vi "fault and error bookkeeping.vi"(0 "data table in":T10, 1 "fault fifo":refnum<k33>, 2 "worker pool reference":T2, 5 "module data":T5={"run state"=enum."sync", "module"=refnum, "module ref"=refnum, "async exec ref"={"command fifo"=refnum, "error fifo"=refnum, "VI Refnum"=refnum, "input buffer"=refnum, "output buffer"=refnum, "process buffer"=refnum, "original dvrs"=[]}, "configuration ref"=refnum, "GUID"={"Hi"=0, "Lo"=0}, "error"={"status"=FALSE, "code"=0, "source"=""}, "previous error code"=0, "input method"={"data table"={"Double"=[], "Single"=[], "I64"=[], "I32"=[], "I16"=[], "I8"=[], "U64"=[], "U32"=[], "U16"=[], "U8"=[], "Boolean"=[], "String"=[], "Array of Double"=[], "Array of Single"=[], "Array of I64"=[], "Array of I32"=[], "Array of I16"=[], "Array of I8"=[], "Array of U64"=[], "Array of U32"=[], "Array of U16"=[], "Array of U8"=[], "Array of Boolean"=[], "Array of String"=[]}, "transfer spec"=[]}, "output method"={"data table"={"Double"=[], "Single"=[], "I64"=[], "I32"=[], "I16"=[], "I8"=[], "U64"=[], "U32"=[], "U16"=[], "U8"=[], "Boolean"=[], "String"=[], "Array of Double"=[], "Array of Single"=[], "Array of I64"=[], "Array of I32"=[], "Array of I16"=[], "Array of I8"=[], "Array of U64"=[], "Array of U32"=[], "Array of U16"=[], "Array of U8"=[], "Array of Boolean"=[], "Array of String"=[]}, "transfer spec"=[]}, "process method parameters"={"data table"={"Double"=[], "Single"=[], "I64"=[], "I32"=[], "I16"=[], "I8"=[], "U64"=[], "U32"=[], "U16"=[], "U8"=[], "Boolean"=[], "String"=[], "Array of Double"=[], "Array of Single"=[], "Array of I64"=[], "Array of I32"=[], "Array of I16"=[], "Array of I8"=[], "Array of U64"=[], "Array of U32"=[], "Array of U16"=[], "Array of U8"=[], "Array of Boolean"=[], "Array of String"=[]}, "transfer spec"=[]}, "process method results"={"data table"={"Double"=[], "Single"=[], "I64"=[], "I32"=[], "I16"=[], "I8"=[], "U64"=[], "U32"=[], "U16"=[], "U8"=[], "Boolean"=[], "String"=[], "Array of Double"=[], "Array of Single"=[], "Array of I64"=[], "Array of I32"=[], "Array of I16"=[], "Array of I8"=[], "Array of U64"=[], "Array of U32"=[], "Array of U16"=[], "Array of U8"=[], "Array of Boolean"=[], "Array of String"=[]}, "transfer spec"=[]}, "fault handling"={"unknown"=[], "trivial"=[], "critical"=[], "recoverable"=[]}, "error report index "=-1} {"GUID"."Lo" format="%.0x"; "GUID"."Hi" format="%.0x"}, 7 "time data in":T1, 9 "run flags in":u8, 11 "engine error in":errorcluster, 12 "module index":i32) -> (4 "data table out":T10, 6 "module data out":T5={"run state"=enum."sync", "module"=refnum, "module ref"=refnum, "async exec ref"={"command fifo"=refnum, "error fifo"=refnum, "VI Refnum"=refnum, "input buffer"=refnum, "output buffer"=refnum, "process buffer"=refnum, "original dvrs"=[]}, "configuration ref"=refnum, "GUID"={"Hi"=0, "Lo"=0}, "error"={"status"=FALSE, "code"=0, "source"=""}, "previous error code"=0, "input method"={"data table"={"Double"=[], "Single"=[], "I64"=[], "I32"=[], "I16"=[], "I8"=[], "U64"=[], "U32"=[], "U16"=[], "U8"=[], "Boolean"=[], "String"=[], "Array of Double"=[], "Array of Single"=[], "Array of I64"=[], "Array of I32"=[], "Array of I16"=[], "Array of I8"=[], "Array of U64"=[], "Array of U32"=[], "Array of U16"=[], "Array of U8"=[], "Array of Boolean"=[], "Array of String"=[]}, "transfer spec"=[]}, "output method"={"data table"={"Double"=[], "Single"=[], "I64"=[], "I32"=[], "I16"=[], "I8"=[], "U64"=[], "U32"=[], "U16"=[], "U8"=[], "Boolean"=[], "String"=[], "Array of Double"=[], "Array of Single"=[], "Array of I64"=[], "Array of I32"=[], "Array of I16"=[], "Array of I8"=[], "Array of U64"=[], "Array of U32"=[], "Array of U16"=[], "Array of U8"=[], "Array of Boolean"=[], "Array of String"=[]}, "transfer spec"=[]}, "process method parameters"={"data table"={"Double"=[], "Single"=[], "I64"=[], "I32"=[], "I16"=[], "I8"=[], "U64"=[], "U32"=[], "U16"=[], "U8"=[], "Boolean"=[], "String"=[], "Array of Double"=[], "Array of Single"=[], "Array of I64"=[], "Array of I32"=[], "Array of I16"=[], "Array of I8"=[], "Array of U64"=[], "Array of U32"=[], "Array of U16"=[], "Array of U8"=[], "Array of Boolean"=[], "Array of String"=[]}, "transfer spec"=[]}, "process method results"={"data table"={"Double"=[], "Single"=[], "I64"=[], "I32"=[], "I16"=[], "I8"=[], "U64"=[], "U32"=[], "U16"=[], "U8"=[], "Boolean"=[], "String"=[], "Array of Double"=[], "Array of Single"=[], "Array of I64"=[], "Array of I32"=[], "Array of I16"=[], "Array of I8"=[], "Array of U64"=[], "Array of U32"=[], "Array of U16"=[], "Array of U8"=[], "Array of Boolean"=[], "Array of String"=[]}, "transfer spec"=[]}, "fault handling"={"unknown"=[], "trivial"=[], "critical"=[], "recoverable"=[]}, "error report index "=-1} {"GUID"."Lo" format="%.0x"; "GUID"."Hi" format="%.0x"}, 8 "safe state?":bool, 10 "run flags out":u8, 15 "engine error out":errorcluster)   [LabVIEW 2013, in "main engine.lvlib"]
uses:
  main engine/main engine.lvlib
  rt fault.ctl
  <vilib>/NI/Tag Bus Module Framework/runtime/error classification.ctl
  <vilib>/NI/Tag Bus Module Framework/module configuration/TBM module configuration.lvclass
  <vilib>/NI/Tag Bus/table/data table.ctl
  full module data.ctl
  <vilib>/NI/Tag Bus Module Framework/runtime/TBM module execution interface.lvclass
  module run state.ctl
  async executor/asynchronous executor reference.ctl
  async executor/message to executor.ctl
  async command notification.ctl
  async error info.ctl
  <vilib>/NI/Configuration Framework/serializable configuration/Numeric GUID.ctl
  module method data.ctl
  <vilib>/NI/Tag Bus/table/transfer specification.ctl
  <vilib>/NI/Tag Bus/tag/Data Type.ctl
  fault handling spec.ctl
  Configuration/Error Actions.ctl
  worker library/worker comms.ctl
  worker library/worker commands.ctl
  worker library/request fifos.ctl
  worker library/recovery request.ctl
  worker library/response fifos.ctl
  worker library/recovery response.ctl
  time information.ctl
  <vilib>/NI/Tag Bus/table/data polymorphs/write one/write I32.vi
  worker library/request recovery.vi
  rt swap object in dvr.vi
  <vilib>/NI/Tag Bus/table/data table.lvlib
  async executor/async executor.lvlib
  <vilib>/NI/Configuration Framework/serializable configuration/NISE_CEF_serializable configuration.lvclass
  Configuration/Standard Engine Configuration.lvclass
  <vilib>/NI/Tag Bus/tag/tag descriptor.lvclass
  worker library/worker pool.lvlib
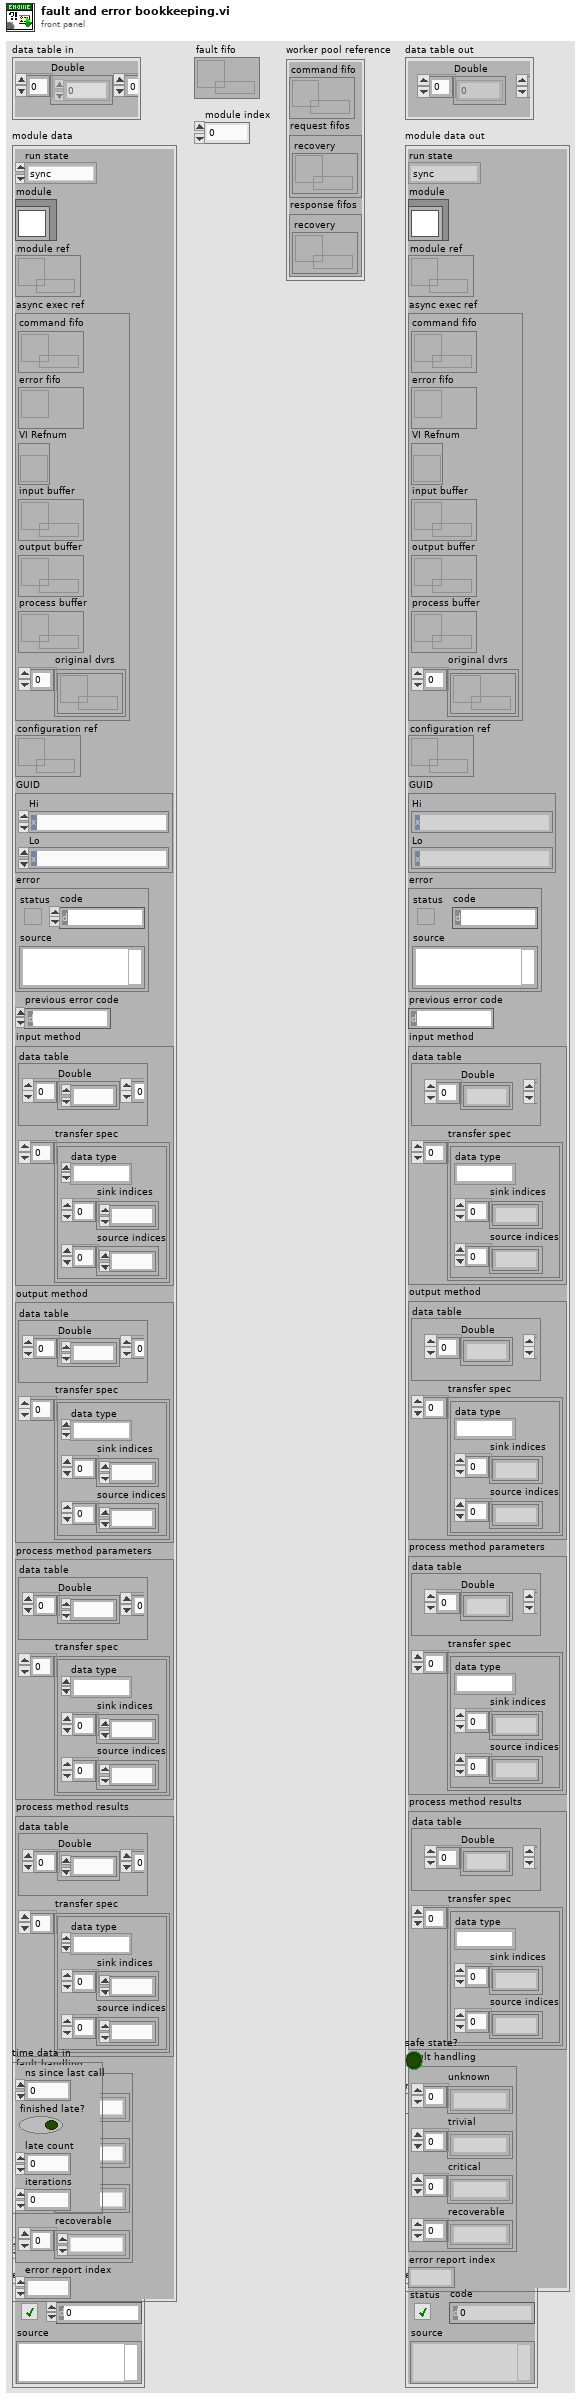
[diagram p1: front panel]
types:
  T1 = typedef "main engine.lvlib/time information.ctl" = cluster{"ns since last call":u64, "finished late?":bool, "late count":u32, "iterations":u64}
  T2 = typedef "worker pool.lvlib/worker comms.ctl" = cluster{"command fifo":refnum<k33>, "request fifos":T3, "response fifos":T4}
  T3 = typedef "worker pool.lvlib/request fifos.ctl" = cluster{"recovery":refnum<k33>}
  T4 = typedef "worker pool.lvlib/response fifos.ctl" = cluster{"recovery":refnum<k33>}
  T5 = typedef "main engine.lvlib/full module data.ctl" = cluster{"run state":T6, "module":refnum<class "TBM module execution interface.lvclass">, "module ref":refnum<data-value>, "async exec ref":T7, "configuration ref":refnum<data-value>, "GUID":T8, "error":errorcluster, "previous error code":i32, "input method":T9, "output method":T9, "process method parameters":T9, "process method results":T9, "fault handling":T13, "error report index ":i32}
  T6 = typedef "main engine.lvlib/module run state.ctl" = enum16{"sync", "async"}
  T7 = typedef "async executor.lvlib/asynchronous executor reference.ctl" = cluster{"command fifo":refnum<k33>, "error fifo":refnum<k33>, "VI Refnum":refnum<vi>, "input buffer":refnum<k33>, "output buffer":refnum<k33>, "process buffer":refnum<k33>, "original dvrs":refnum<data-value>[]}
  T8 = typedef "NISE_CEF_serializable configuration.lvclass/Numeric GUID.ctl" = cluster{"Hi":u64, "Lo":u64}
  T9 = typedef "main engine.lvlib/module method data.ctl" = cluster{"data table":T10, "transfer spec":T11[]}
  T10 = typedef "tag bus.lvlib/data table.lvlib/data table.ctl" = cluster{"Double":dbl[], "Single":sgl[], "I64":i64[], "I32":i32[], "I16":i16[], "I8":i8[], "U64":u64[], "U32":u32[], "U16":u16[], "U8":u8[], "Boolean":bool[], "String":string[], "Array of Double":cluster{"DBL Array":dbl[]}[], "Array of Single":cluster{"SGL Array":sgl[]}[], "Array of I64":cluster{"I64 Array":i64[]}[], "Array of I32":cluster{"I32 Array":i32[]}[], "Array of I16":cluster{"I16 Array":i16[]}[], "Array of I8":cluster{"I8 Array":i8[]}[], "Array of U64":cluster{"U64 Array":u64[]}[], "Array of U32":cluster{"U32 Array":u32[]}[], "Array of U16":cluster{"U16 Array":u16[]}[], "Array of U8":cluster{"U8 Array":u8[]}[], "Array of Boolean":cluster{"Boolean Array":bool[]}[], "Array of String":cluster{"String Array":string[]}[]}
  T11 = typedef "tag bus.lvlib/data table.lvlib/transfer specification.ctl" = cluster{"data type":T12, "sink indices":i32[], "source indices":i32[]}
  T12 = typedef "tag bus.lvlib/tag descriptor.lvclass/Data Type.ctl" = enum16{"Double", "Single", "I64", "I32", "I16", "I8", "U64", "U32", "U16", "U8", "Boolean", "String", "Array of Double", "Array of Single", "Array of I64", "Array of I32", "Array of I16", "Array of I8", "Array of U64", "Array of U32", "Array of U16", "Array of U8", "Array of Boolean", "Array of String"}
  T13 = typedef "main engine.lvlib/fault handling spec.ctl" = cluster{"unknown":T14[], "trivial":T14[], "critical":T14[], "recoverable":T14[]}
  T14 = typedef "Standard Engine Configuration.lvclass/Error Actions.ctl" = enum16{"Clear", "Notify", "Stop Component", "Stop Engine", "Safe State", "Attempt Recovery"}
  T15 = typedef "TBM module execution interface.lvclass/error classification.ctl" = enum16{"unknown", "none", "trivial", "recoverable", "critical"}
  T16 = typedef "async executor.lvlib/async error info.ctl" = cluster{"error code":i32, "error classification":T15}
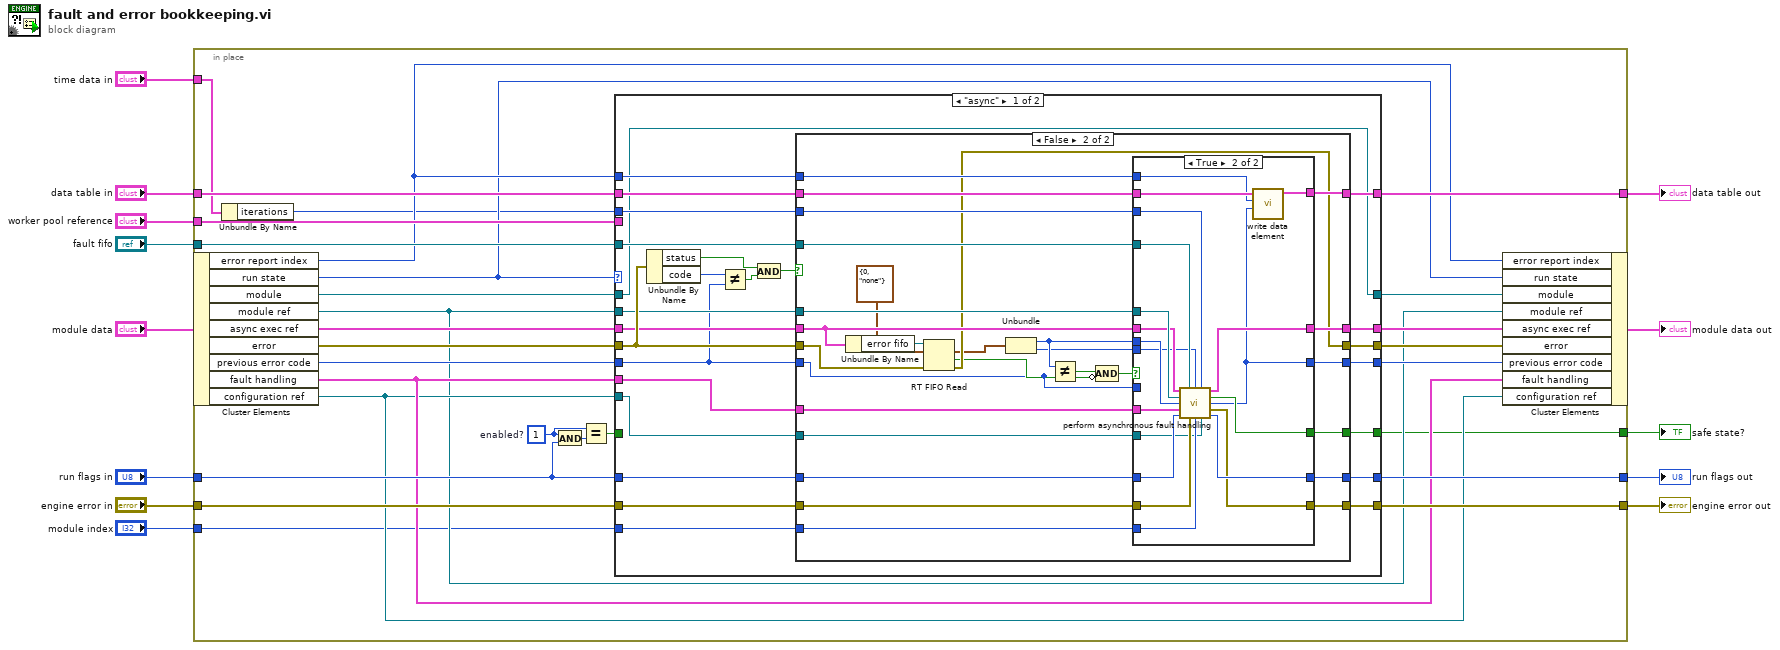
[diagram p0: block diagram]
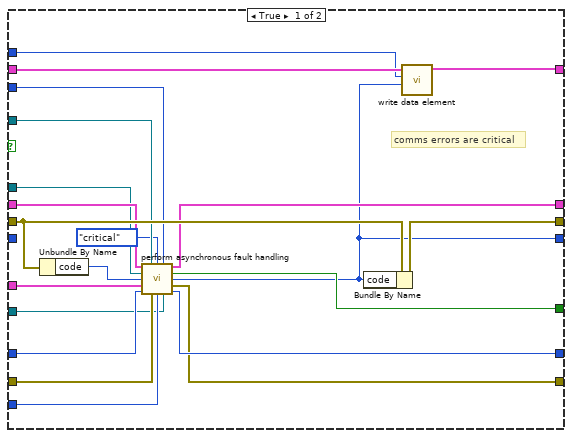
[diagram p2: hidden frame]
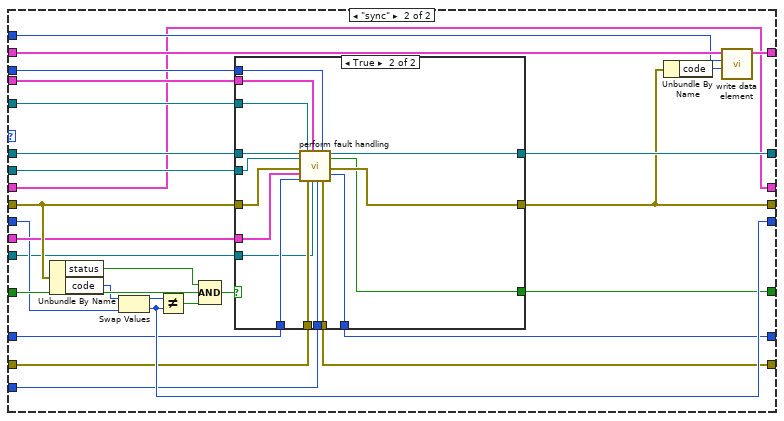
[diagram p4: hidden frame]
diagram:
  n1 = in-place {
    in-place-border: [w41] -> w13
    in-place-border: "run flags in" -> [w40]
    in-place-border: "fault fifo" -> [w39]
    in-place-border: [w35] -> w10
    in-place-border: "data table in" -> [w34]
    in-place-border: "engine error in" -> [w33]
    in-place-border: [w32] -> w7
    in-place-border: "worker pool reference" -> [w31]
    in-place-border: "time data in" -> [w17]
    in-place-border: "module index" -> [w16]
    in-place-border: [w14] -> w1
    w37 = u8 1  # enabled?
    n2 = in-place-cluster #1("module data") -> ("error report index"=w30:i32, "run state"=w29:T6, "module"=w28:refnum<class "TBM module execution interface.lvclass">, "module ref"=w18:refnum<data-value>, "async exec ref"=w27:T7, "error"=w26:errorcluster, "previous error code"=w25:i32, "fault handling"=w20:T13, "configuration ref"=w19:refnum<data-value>)
    n3 = Unbundle By Name(w17) -> ("iterations"=w15:u64)
    n4 = And(x=w37, y=w40) -> (x .and. y?=w36:u8)
    n5 = Equal?(x=w37, y=w36) -> (x = y?=w38:bool)
    n6 = case shown="\"async\"" w29 {
      tunnel: w34 -> [w65 w168]
      tunnel: [w64 w167] -> w35
      tunnel: w30 -> [w63 w166]
      tunnel: w38 -> [_ w165]
      tunnel: w28 -> [w42 w163]
      tunnel: [w42 w162] -> w21
      tunnel: [w59 w140] -> w22
      tunnel: w27 -> [w60 w140]
      tunnel: w26 -> [w61 w161]
      tunnel: w20 -> [w47 w160]
      tunnel: [w62 w150] -> w23
      tunnel: w18 -> [w50 w158]
      tunnel: w39 -> [w52 w157]
      tunnel: w25 -> [w43 w153]
      tunnel: [w58 w152] -> w24
      tunnel: [w57 w148] -> w41
      tunnel: w40 -> [w56 w149]
      tunnel: w33 -> [w55 w147]
      tunnel: [w49 w146] -> w32
      tunnel: w31 -> [_ w143]
      tunnel: w19 -> [w48 w145]
      tunnel: w16 -> [w54 w144]
      tunnel: w15 -> [w51 w142]
      tunnel: [w53 w141] -> w14
      frame "async" {
        n7 = Unbundle By Name(w61) -> ("status"=w66:bool, "code"=w44:i32)
        n8 = Not Equal?(x=w44, y=w43) -> (x != y?=w45:bool)
        n9 = And(x=w66, y=w45) -> (x .and. y?=w46:bool)
        n10 = case shown="False" w46 {
          tunnel: w65 -> [w86 w114]
          tunnel: [w87 w115] -> w64
          tunnel: w63 -> [w85 w113]
          tunnel: [w73 w97] -> w62
          tunnel: w61 -> [w84 w112]
          tunnel: w60 -> [w77 w98]
          tunnel: [w78 w106] -> w59
          tunnel: [w68 w99] -> w58
          tunnel: [w81 w109] -> w57
          tunnel: w56 -> [w80 w108]
          tunnel: w55 -> [w83 w111]
          tunnel: w54 -> [w82 w110]
          tunnel: [w79 w107] -> w53
          tunnel: w52 -> [w76 w105]
          tunnel: w51 -> [w75 w104]
          tunnel: w50 -> [w72 w103]
          tunnel: [w71 w102] -> w49
          tunnel: w48 -> [w70 w101]
          tunnel: w47 -> [w69 w100]
          tunnel: w43 -> [_ w92]
          frame True {
            # "comms errors are critical"
            n11 = Unbundle By Name(w84) -> ("code"=w74:i32)
            n12 = call "perform asynchronous fault handling.vi"("module in"=w77, "fault fifo"=w76, "error classification"=error_classification."critical", "iteration"=w75, "module ref in"=w72, "code"=w74, "fault handling in"=w69, "run flags in"=w80, "engine error in"=w83, "engine reference"=w82, "cfg ref"=w70) -> ("module out"=w78:T7, "go to safe state"=w79:bool, "code out"=w68:i32, "engine error out"=w71:errorcluster, "run flags out"=w81:u8)
            n13 = Bundle By Name(cluster=w84, "code"=w68) -> (w73:errorcluster)
            n14 = call-poly <vilib>:"write data element.vi"("value"=w68, "index"=w85, "data table in"=w86) -> ("data table out"=w87:T10)  [unwired: 8 in]
          }
          frame False {
            n15 = Unbundle By Name(w98) -> ("error fifo"=w96:refnum<k33>)
            n16 = RT FIFO Read(0:w96, 1:T16 {"error code"=0, "error classification"=enum."none"} ("element"), 3:w112) -> (9:w93:T16, 10:w95:bool, 11:w97:errorcluster)  [unwired: 1 in, 2 out]
            n17 = Unbundle(w93) -> ("error code"=w91:i32, "error classification"=w89:T15)
            n18 = Not Equal?(x=w91, y=w92) -> (x != y?=w90:bool)
            n19 = Compound Arithmetic op=AND(w90, invert w95) -> (w94:bool)
            n20 = case shown="True" w94 {
              tunnel: [w120 w139] -> w115
              tunnel: w114 -> [w120 w138]
              tunnel: w113 -> [_ w137]
              tunnel: w111 -> [w116 w136]
              tunnel: w110 -> [_ w135]
              tunnel: [w117 w134] -> w109
              tunnel: w108 -> [w117 w133]
              tunnel: [_ w132] -> w107
              tunnel: [w119 w131] -> w106
              tunnel: w105 -> [_ w130]
              tunnel: w104 -> [_ w129]
              tunnel: w103 -> [_ w128]
              tunnel: [w116 w127] -> w102
              tunnel: w101 -> [_ w126]
              tunnel: w100 -> [_ w125]
              tunnel: [w118 w124] -> w99
              tunnel: w98 -> [w119 w123]
              tunnel: w92 -> [w118 _]
              tunnel: w91 -> [_ w122]
              tunnel: w89 -> [_ w121]
              frame False {
              }
              frame True {
                n21 = call "perform asynchronous fault handling.vi"("module in"=w123, "fault fifo"=w130, "error classification"=w121, "iteration"=w129, "module ref in"=w128, "code"=w122, "fault handling in"=w125, "run flags in"=w133, "engine error in"=w136, "engine reference"=w135, "cfg ref"=w126) -> ("module out"=w131:T7, "go to safe state"=w132:bool, "code out"=w124:i32, "engine error out"=w127:errorcluster, "run flags out"=w134:u8)
                n22 = call-poly <vilib>:"write data element.vi"("value"=w124, "index"=w137, "data table in"=w138) -> ("data table out"=w139:T10)  [unwired: 8 in]
              }
            }
          }
        }
      }
      frame "sync" {
        n23 = Unbundle By Name(w161) -> ("status"=w159:bool, "code"=w154:i32)
        n24 = Swap Values(12:w154, 14:w153) -> (1:w155:i32, 3:w152:i32)  [unwired: 1 in]
        n25 = Not Equal?(x=w155, y=w152) -> (x != y?=w156:bool)
        n26 = Compound Arithmetic op=AND(w159, w165, w156) -> (w164:bool)
        n27 = case shown="True" w164 {
          tunnel: w163 -> [w172 w187]
          tunnel: [w172 w188] -> w162
          tunnel: w161 -> [w171 w183]
          tunnel: [w171 w185] -> w150
          tunnel: w160 -> [_ w184]
          tunnel: w158 -> [_ w186]
          tunnel: w157 -> [_ w180]
          tunnel: w149 -> [w170 w182]
          tunnel: [w170 w181] -> w148
          tunnel: w147 -> [w169 w179]
          tunnel: [w169 w178] -> w146
          tunnel: w145 -> [_ w177]
          tunnel: w144 -> [_ w176]
          tunnel: w143 -> [_ w175]
          tunnel: w142 -> [_ w174]
          tunnel: [_ w173] -> w141
          frame False {
          }
          frame True {
            n28 = call "perform fault handling.vi"("module in"=w187, "module ref in"=w186, "error in"=w183, "fault handling in"=w184, "run flags in"=w182, "fault fifo"=w180, "engine error in"=w179, "worker pool in"=w175, "cfg ref"=w177, "engine reference"=w176, "iteration"=w174) -> ("engine error out"=w178:errorcluster, "module out"=w188:refnum<class "TBM module execution interface.lvclass">, "go to safe state"=w173:bool, "error out"=w185:errorcluster, "run flags out"=w181:u8)  [unwired: 4 in]
          }
        }
        n29 = Unbundle By Name(w150) -> ("code"=w151:i32)
        n30 = call-poly <vilib>:"write data element.vi"("value"=w151, "index"=w166, "data table in"=w168) -> ("data table out"=w167:T10)  [unwired: 8 in]
      }
    }
    n31 = in-place-cluster #1("error report index"=w30, "run state"=w29, "module"=w21, "module ref"=w18, "async exec ref"=w22, "error"=w23, "previous error code"=w24, "fault handling"=w20, "configuration ref"=w19) -> (→"module data out":T5)
  }
  "run flags out" <- w13
  "data table out" <- w10
  "engine error out" <- w7
  "safe state?" <- w1
